vi "Grid KeyDown BoolCol.vi"(4 "表サイズ(縦×横)":i32[](array[numeric]), 6 "EditPos":T1, 8 "error in (no error)":errorcluster caption="エラー入力（エラーなし）", 9 "Char":i16, 10 "ref.表":refnum<vi>, 11 "Control入力":refnum<vi>) -> (0 "error out":errorcluster caption="エラー出力", 1 "セル文字列":string, 3 "ブール":bool)   [LabVIEW 2014]
uses:
  <vilib>/event_ctls.llb/eventvkey.ctl
  <vilib>/Utility/miscctls.llb/LVRowAndColumnTypeDef.ctl
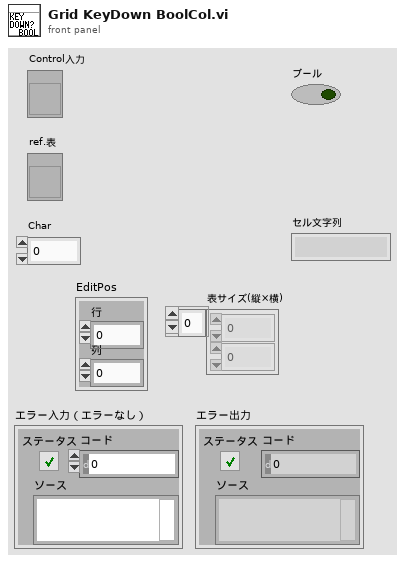
[diagram p1: front panel]
types:
  T1 = typedef "LVRowAndColumnTypeDef.ctl" = cluster{"Row":i32, "Column":i32}
  T2 = typedef "eventvkey.ctl" = enum16{"ASCII", "Enter", "Return", "Shift", "Ctrl", "Alt", "Cmd", "Opt", "Caps", "NumLock", "Clear", "Break", "Up", "Down", "Left", "Right", "Insert", "Delete", "Home", "End", "PageUp", "PageDown", "Escape", "Help", "Pause", "ScrollLock", "F1", "F2", "F3", "F4", "F5", "F6", "F7", "F8", "F9", "F10", "F11", "F12", "F13", "F14", "F15", "F16", "F17", "F18", "F19", "F20", "F21", "F22", "F23", "F24", "Play", "VolumeUp", "VolumeDown", "Mute", "Two Byte Char"}
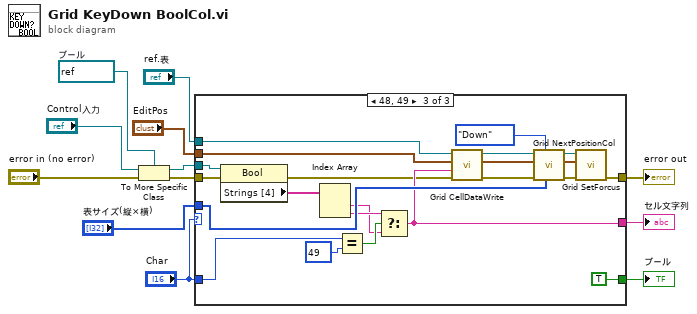
[diagram p0: block diagram]
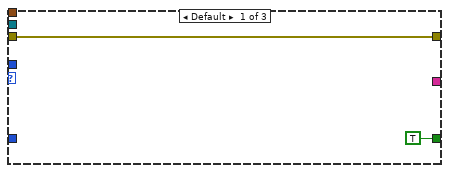
[diagram p2: hidden frame]
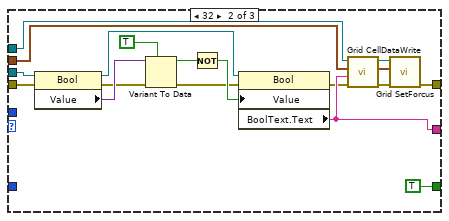
[diagram p3: hidden frame]
diagram:
  w6 = refnum<vi> refnum  # ブール
  n1 = To More Specific Class(target class=w6, reference="Control入力", error in="error in (no error)") -> (specific class reference=w8:refnum<vi>, error out=w2:errorcluster)
  n2 = case shown="48, 49" "Char" {
    tunnel: "Char" -> [_ _ w53]
    tunnel: "表サイズ(縦×横)" -> [_ _ w51]
    tunnel: w8 -> [_ w32 w49]
    tunnel: "ref.表" -> [_ w26 w48]
    tunnel: "EditPos" -> [_ w25 w47]
    tunnel: [TRUE TRUE TRUE] -> w12
    tunnel: [_ w20 w36] -> w4
    tunnel: w2 -> [w13 w15 w35]
    tunnel: [w13 w19 w33] -> w1
    frame Default {
    }
    frame 32 {
      n3 = property class="Bool"(reference=w32, error in=w15) -> (reference out=w28:refnum<vi>, error out=w16:errorcluster, "Value"=w30:variant)
      n4 = Variant To Data(error in=w16, type=TRUE, Variant=w30) -> (data=w29:bool, error out=w17:errorcluster)
      n5 = Not(x=w29) -> (.not. x?=w27:bool)
      n6 = property class="Bool"(reference=w28, error in=w17, "Value"=w27) -> (error out=w18:errorcluster, "BoolText.Text"=w20:string)  [unwired: 1 out]
      n7 = call "Grid CellDataWrite.vi"("error in (no error)"=w18, "RingText.Text"=w20, "EditPos"=w25, "Table入力"=w26) -> ("エラー出力"=w22:errorcluster, "EditPos(copy))"=w24:T1, "Table出力"=w23:refnum<vi>)  [unwired: 5 in]
      n8 = call "Grid SetForcus.vi"("エラー入力（エラーなし）"=w22, "EditPos入力"=w24, "Table入力"=w23) -> ("error out"=w19:errorcluster)  [unwired: 6 in, 2 out]
    }
    frame 48, 49 {
      n9 = property class="Bool"(reference=w49, error in=w35) -> (error out=w34:errorcluster, "Strings [4]"=w50:string[])  [unwired: 1 out]
      n10 = Index Array(array=w50) -> (element #1=w38:string, element #2=w39:string)  [unwired: 2 in]
      n11 = Equal?(x=w53, y=i16 49) -> (x = y?=w52:bool)
      n12 = Select(t=w39, s=w52, f=w38) -> (s? t:f=w36:string)
      n13 = call "Grid CellDataWrite.vi"("error in (no error)"=w34, "RingText.Text"=w36, "EditPos"=w47, "Table入力"=w48) -> ("エラー出力"=w41:errorcluster, "EditPos(copy))"=w46:T1, "Table出力"=w43:refnum<vi>)  [unwired: 5 in]
      n14 = call "Grid NextPositionCol.vi"("表サイズ(縦x横)"=w51, "VKey(Right)"=eventvkey."Down" ("VKey"), "error in (no error)"=w41, "EditPos入力"=w46, "ref.表"=w43) -> ("error out"=w40:errorcluster, "EditPos出力"=w45:T1, "ref.表(copy)"=w42:refnum<vi>)  [unwired: 4 in]
      n15 = call "Grid SetForcus.vi"("エラー入力（エラーなし）"=w40, "EditPos入力"=w45, "Table入力"=w42) -> ("error out"=w33:errorcluster)  [unwired: 6 in, 2 out]
    }
  }
  "ブール" <- w12
  "error out" <- w1
  "セル文字列" <- w4
